vi "BSC203ConnectMoveTo.vi"() -> ()   [LabVIEW 2023]
uses:
  C:/Users/fmovagharnemati/OneDrive - THORLABS Inc/Desktop/github/BSC203/Thorlabs.MotionControl.Controls.dll
  Thorlabs.MotionControl.Controls.dll
  C:/Users/fmovagharnemati/OneDrive - THORLABS Inc/Desktop/github/BSC203/Thorlabs.MotionControl.Benchtop.StepperMotorCLI.dll
  Thorlabs.MotionControl.Benchtop.StepperMotorCLI.dll
panel:
  in  "Channel 3":refnum<k24>(container)
  in  "Channel 2":refnum<k24>(container)
  in  "?":bool
  in  "Set Abs Pos":bool
  in  "MoveAbsolute":bool
  in  "Home":bool
  in  "Abs Pos":dbl
  in  "Relative Move":bool
  in  "direction":i32(ring)=1 items=["Forward"=1, "Backward"=2]
  in  "Step Size":dbl
  in  "SerialNumber":string
  in  "Channel 1":refnum<k24>(container)
  # "Thorlabs Hardware: BSC203 -Benchtop Stepper Motor Controllers\nhttps://www.thorlabs.com/thorproduct.cfm?partnumber=BSC203\n\nDescription: This VI will enable you to communicate with BSC203 series to control stepper motors. This example enables all 3 channels, but only channel 1 is wired to move commands. \n\nInstructions: \n1) Connect your BSC203 device to your PC & power the device, ensuring your stage/actutator is connected. For full device setup, the device product manual can be found on our website.\n2) Enter the device serial number below.\n3) Click 'Run' in the LabVIEW Toolbar which will attempt a connection, and enable the device.\n4) Ensure the device move path is clear for homing, and press Home.\n5) Await for device to be be available, and to have finished homing (Home indicator in control panel should be green).\n6) Input desired absolute position, and press 'Set Abs Pos' to set that for absolute moves.\n7) Similarly input desired direction and step size for relative moves.\n8) To end the Program click 'STOP'."
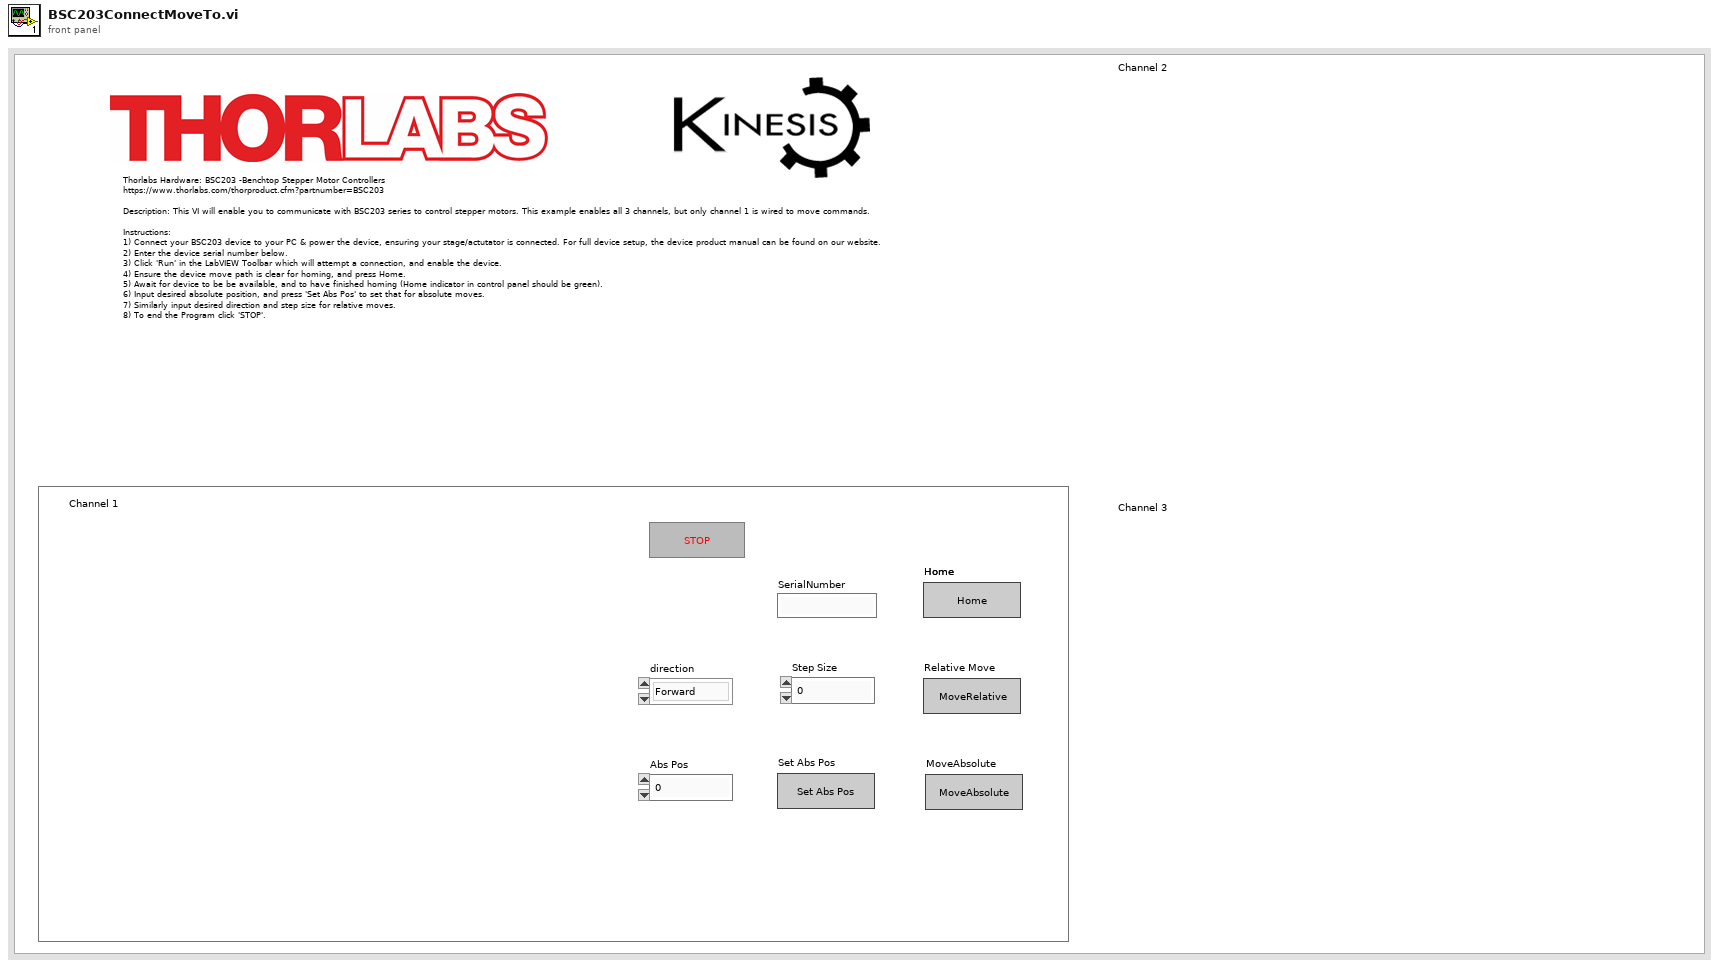
[diagram p1: front panel]
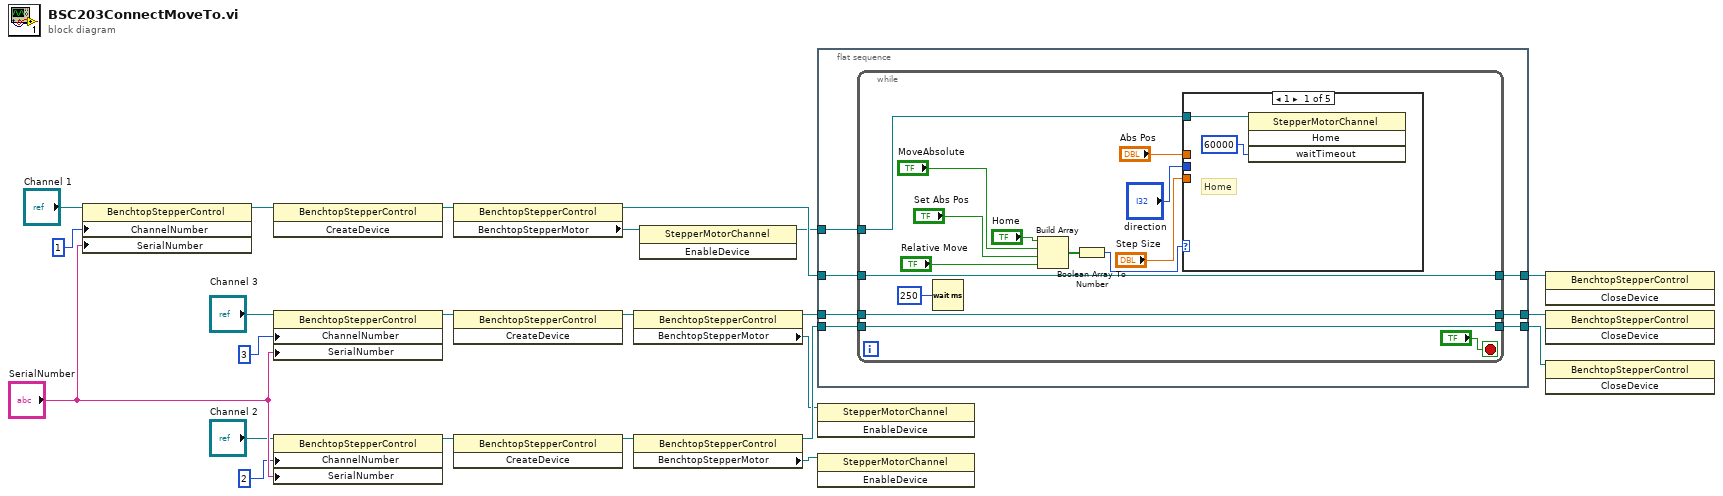
[diagram p0: block diagram]
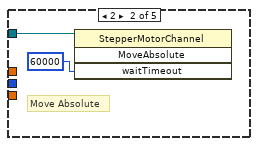
[diagram p2: hidden frame]
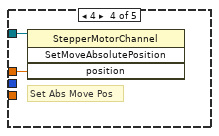
[diagram p4: hidden frame]
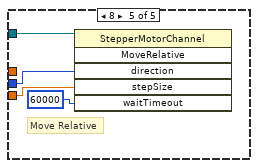
[diagram p5: hidden frame]
diagram:
  n1 = property class="BenchtopStepperControl"(reference="Channel 1", "ChannelNumber"=1, "SerialNumber"="SerialNumber") -> (reference out=w21:refnum<k24>)  [unwired: 1 in, 1 out]
  n2 = invoke class="BenchtopStepperControl" method="CreateDevice"(reference=w21) -> (reference out=w20:refnum<k24>)  [unwired: 2 in, 2 out]
  n3 = property class="BenchtopStepperControl"(reference="Channel 3", "ChannelNumber"=3, "SerialNumber"="SerialNumber") -> (reference out=w8:refnum<k24>)  [unwired: 1 in, 1 out]
  n4 = property class="BenchtopStepperControl"(reference="Channel 2", "ChannelNumber"=2, "SerialNumber"="SerialNumber") -> (reference out=w9:refnum<k24>)  [unwired: 1 in, 1 out]
  n5 = property class="BenchtopStepperControl"(reference=w20) -> (reference out=w19:refnum<k24>, "BenchtopStepperMotor"=w17:refnum<k24>)  [unwired: 1 in, 1 out]
  n6 = invoke class="BenchtopStepperControl" method="CreateDevice"(reference=w8) -> (reference out=w6:refnum<k24>)  [unwired: 2 in, 2 out]
  n7 = invoke class="BenchtopStepperControl" method="CreateDevice"(reference=w9) -> (reference out=w7:refnum<k24>)  [unwired: 2 in, 2 out]
  n8 = property class="BenchtopStepperControl"(reference=w6) -> (reference out=w12:refnum<k24>, "BenchtopStepperMotor"=w10:refnum<k24>)  [unwired: 1 in, 1 out]
  n9 = property class="BenchtopStepperControl"(reference=w7) -> (reference out=w13:refnum<k24>, "BenchtopStepperMotor"=w11:refnum<k24>)  [unwired: 1 in, 1 out]
  n10 = invoke class="StepperMotorChannel" method="EnableDevice"(reference=w17) -> (reference out=w16:refnum<k24>)  [unwired: 2 in, 2 out]
  n11 = flat-sequence {
    tunnel: w19 -> [w30]
    tunnel: [w29] -> w18
    tunnel: w16 -> [w28]
    tunnel: [w27] -> w15
    tunnel: [w25] -> w14
    tunnel: w13 -> [w26]
    tunnel: w12 -> [w24]
    frame #0 {
      n12 = while {
        tunnel: [w37] -> w29
        tunnel: w28 -> [w41]
        tunnel: w30 -> [w37]
        tunnel: [w32] -> w27
        tunnel: w26 -> [w32]
        tunnel: [w31] -> w25
        tunnel: w24 -> [w31]
        stop <- "?" stop-if-true
        n13 = Wait (ms)(milliseconds to wait=u32 250) -> ()  [unwired: 1 out]
        n14 = Build Array("Home", "MoveAbsolute", "Set Abs Pos", "Relative Move") -> (w40:bool[])
        n15 = Boolean Array To Number(Boolean array=w40) -> (number=w39:u32)
        n16 = case shown="1" w39 {
          tunnel: w41 -> [w46 w48 _ w50 w53]
          tunnel: "Abs Pos" -> [_ _ _ w51 _]
          tunnel: "direction" -> [_ _ _ _ w54]
          tunnel: "Step Size" -> [_ _ _ _ w55]
          frame 1 {
            # "Home"
            n17 = invoke class="StepperMotorChannel" method="Home"(reference=w46, "waitTimeout"=60000) -> ()  [unwired: 2 in, 4 out]
          }
          frame 2 {
            # "Move Absolute"
            n18 = invoke class="StepperMotorChannel" method="MoveAbsolute"(reference=w48, "waitTimeout"=60000) -> ()  [unwired: 2 in, 4 out]
          }
          frame Default {
          }
          frame 4 {
            # "Set Abs Move Pos"
            n19 = invoke class="StepperMotorChannel" method="SetMoveAbsolutePosition"(reference=w50, "position"=w51) -> ()  [unwired: 2 in, 4 out]
          }
          frame 8 {
            # "Move Relative"
            n20 = invoke class="StepperMotorChannel" method="MoveRelative"(reference=w53, "direction"=w54, "stepSize"=w55, "waitTimeout"=60000) -> ()  [unwired: 2 in, 6 out]
          }
        }
      }
    }
  }
  n21 = invoke class="StepperMotorChannel" method="EnableDevice"(reference=w10) -> ()  [unwired: 2 in, 3 out]
  n22 = invoke class="StepperMotorChannel" method="EnableDevice"(reference=w11) -> ()  [unwired: 2 in, 3 out]
  n23 = invoke class="BenchtopStepperControl" method="CloseDevice"(reference=w18) -> ()  [unwired: 2 in, 3 out]
  n24 = invoke class="BenchtopStepperControl" method="CloseDevice"(reference=w14) -> ()  [unwired: 2 in, 3 out]
  n25 = invoke class="BenchtopStepperControl" method="CloseDevice"(reference=w15) -> ()  [unwired: 2 in, 3 out]
